vi "PM9 Set Temp and Wait.vi"(0 "VISA":refnum<visa-resource-name>="TCPIP0::169.254.70.190::502::SOCKET", 5 "Error In":errorcluster, 6 "Accuracy +/-":dbl=0.25 format="%.3g", 7 "Set Point":dbl=25.0 format="%.3g", 9 "RO(t)":bool, 11 "Min (-1 for cont.)":dbl, 12 "Refresh Rate(s)":dbl format="%#_13g", 13 "close session(t)":bool=TRUE) -> (10 "temp":sgl[](array[numeric])=[24.988047, 24.909956], 14 "visa":refnum<visa-resource-name>="TCPIP0::169.254.70.190::502::SOCKET", 15 "session out":refnum<k24>, 19 "error out":errorcluster)   [LabVIEW 2018]
uses:
  C:/RageATE-Tetra/Instruments/Ess Temp Plate/LabView Driver/Public/Watbus.dll
  Public/Watbus.dll
panel:
  out "read_loop(t)":bool
  out "sec":i32
  out "x/y":dbl
  out "vi called (t)":bool
  out "call chain":string[](array[string])
  out "soak(f)":bool=TRUE
  out "elapsed(s)":i32
  out "start":dbl=15892.4205274 format="%_19f"
  in  "Stop":bool
  out "LSL":dbl=24.75
  out "USL":dbl=25.25
  in  "deviceType":i32(ring) items=["Controller", "RUI", "PC", "CommsCard"]
  in  "InstanceId":i32=1
  in  "Zone":i32=1
  in  "TemperatureUnits":i16(ring) items=["Degrees C", "Degrees F"]
  out "Waveform Chart 3":cluster{"Value":sgl, "Value":sgl}(graph)={"Value"=24.988047, "Value"=24.909956}
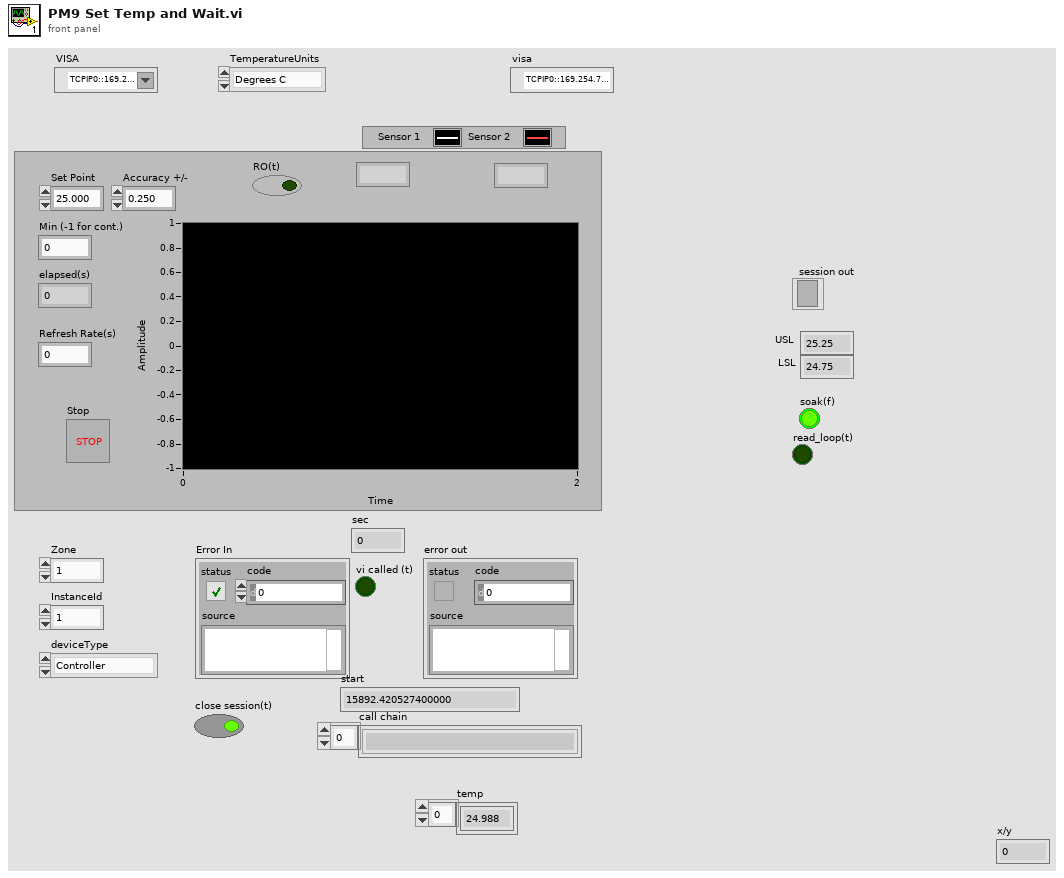
[diagram p1: front panel]
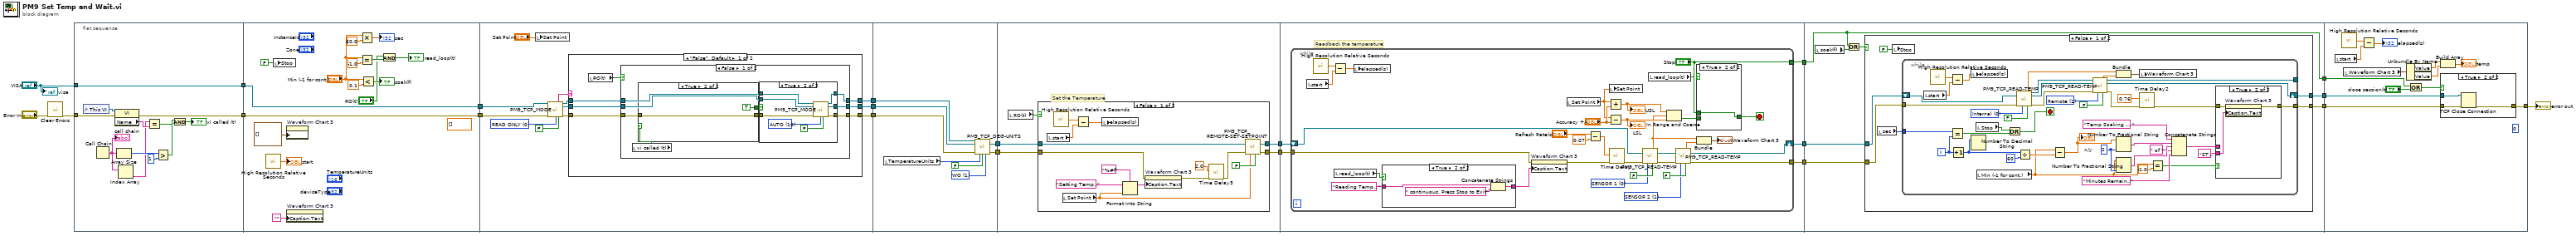
[diagram p0: block diagram]
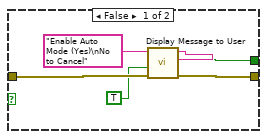
[diagram p2: hidden frame]
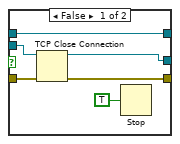
[diagram p3: hidden frame]
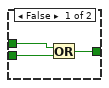
[diagram p8: hidden frame]
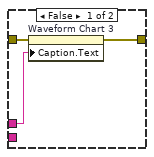
[diagram p9: hidden frame]
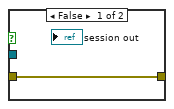
[diagram p11: hidden frame]
diagram:
  n1 = call <vilib>:"Clear Errors.vi"("error in (no error)"="Error In") -> ("error out"=w4:errorcluster)  [unwired: 5 in, 1 out]
  n2 = flat-sequence {
    tunnel: w4 -> [w23]
    tunnel: "VISA" -> [w33]
    tunnel: [w33] -> w2
    tunnel: [w22] -> w1
    tunnel: [w48] -> w15
    tunnel: [w47] -> w14
    tunnel: w2 -> [w48]
    tunnel: w1 -> [w47]
    tunnel: [w51] -> w17
    tunnel: [w57] -> w16
    tunnel: w15 -> [w56]
    tunnel: w14 -> [w59]
    tunnel: [w52] -> w6
    tunnel: [w108] -> w19
    tunnel: [w109] -> w18
    tunnel: w17 -> [w111]
    tunnel: w16 -> [w110]
    tunnel: w6 -> [w104]
    tunnel: [w114] -> w21
    tunnel: [w113] -> w20
    tunnel: w19 -> [w116]
    tunnel: w18 -> [w115]
    tunnel: [w136] -> w13
    tunnel: w21 -> [w138]
    tunnel: w20 -> [w137]
    tunnel: [w135] -> w10
    tunnel: [w134] -> w8
    tunnel: w13 -> [w182]
    tunnel: [w181] -> w12
    tunnel: [w185] -> w11
    tunnel: w10 -> [w183]
    tunnel: [w183] -> w9
    tunnel: w8 -> [w184]
    tunnel: w12 -> [w253]
    tunnel: w11 -> [w249]
    tunnel: w9 -> [w250]
    tunnel: [w241] -> w3
    frame #0 {
      n3 = control-ref of="This VI"() -> (w25:refnum<vi>)
      n4 = Call Chain() -> (call chain=w28:string[])
      "call chain" <- w28
      n5 = property class="VI"(reference=w25, error in=w23) -> (error out=w22:errorcluster, "Name"=w27:string)  [unwired: 1 out]
      n6 = Array Size(array=w28) -> (size(s)=w29:i32)
      n7 = Index Array(array=w28) -> (element=w26:string)  [unwired: 1 in]
      n8 = Equal?(x=w26, y=w27) -> (x = y?=w30:bool)
      n9 = Greater?(x=w29, y=1) -> (0:w31:bool)
      n10 = And(x=w31, y=w30) -> (x .and. y?=→"vi called (t)":bool)
    }
    frame #1 {
      (unwired) dbl[] [] ("History Data")
      n11 = call <vilib>:"High Resolution Relative Seconds.vi"() -> ("relative seconds"=→"start":dbl)
      n12 = local write "Stop"(FALSE ("Stop")) -> ()
      n13 = property on="Waveform Chart 3" class="WFChart (strict)"("History Data"=cluster{"Value":sgl, "Value":sgl}[] []) -> ()  [unwired: 2 in, 2 out]
      n14 = property on="Waveform Chart 3" class="WFChart (strict)"("Caption.Text"="") -> ()  [unwired: 2 in, 2 out]
      n15 = Multiply(x="Min (-1 for cont.)", y=60.0) -> (x*y=→"sec":dbl)
      n16 = Equal?(x="Min (-1 for cont.)", y=-1.0) -> (x = y?=w37:bool)
      n17 = Less?(x="Min (-1 for cont.)", y=0.1) -> (x < y?=→"soak(f)":bool)
      n18 = And(x="RO(t)", y=w37) -> (x .and. y?=→"read_loop(t)":bool)
    }
    frame #2 {
      w54 = u16 0 items=["READ ONLY"=0, "AUTO"=10, "OFF"=62, "MAN"=54] ("MODE")
      n19 = local write "Set Point"("Set Point") -> ()
      n20 = call "PM9_TCP_MODE.vi"("VISA"=w56, "error in (no error)"=w59, "MODE"=w54, "Close tcp(t)"=FALSE) -> ("mode(read)"=w49:string, "visa out"=w50:refnum<visa-resource-name>, "connection ID out"=w53:refnum<k5>, "error out"=w58:errorcluster)  [unwired: 8 in]
      n21 = case shown="\"False\", Default" w49 {
        tunnel: w58 -> [w67 w103]
        tunnel: [w66 w103] -> w57
        tunnel: w53 -> [w65 w102]
        tunnel: [w64 w102] -> w52
        tunnel: [w62 w101] -> w51
        tunnel: w50 -> [w63 w101]
        frame "False", Default {
          n22 = local read "RO(t)"() -> (w61:bool)
          n23 = case shown="False" w61 {
            tunnel: w67 -> [w76 w98]
            tunnel: [w74 w98] -> w66
            tunnel: w65 -> [w72 w99]
            tunnel: [w71 w99] -> w64
            tunnel: w63 -> [w70 w100]
            tunnel: [w69 w100] -> w62
            frame False {
              n24 = local read "vi called (t)"() -> (w68:bool)
              n25 = case shown="True" w68 {
                tunnel: w76 -> [w81 w82]
                tunnel: [w78 TRUE ("OK")] -> w75
                tunnel: [w77 w82] -> w73
                frame False {
                  n26 = call "Display Message to User"("error in (no error)"=w81, "Enable"=TRUE, "Message"="Enable Auto Mode (Yes)\nNo to Cancel") -> ("error out"=w77:errorcluster, "OK"=w78:bool)  [unwired: 7 in]
                }
                frame True {
                }
              }
              n27 = case shown="True" w75 {
                tunnel: [w86 w97] -> w74
                tunnel: w73 -> [w87 w96]
                tunnel: w72 -> [w88 w94]
                tunnel: [w84 w93] -> w71
                tunnel: w70 -> [w89 w92]
                tunnel: [w89 w91] -> w69
                frame False {
                  n28 = TCP Close Connection(connection ID=w88, error in (no error)=w87) -> (connection ID out=w84:refnum<k5>, error out=w86:errorcluster)  [unwired: 1 in]
                  n29 = Stop(stop? (T)=TRUE) -> ()
                }
                frame True {
                  w95 = u16 10 items=["READ ONLY"=0, "AUTO"=10, "OFF"=62, "MAN"=54] ("MODE")
                  n30 = call "PM9_TCP_MODE.vi"("VISA"=w92, "connection ID"=w94, "error in (no error)"=w96, "MODE"=w95, "Close tcp(t)"=FALSE) -> ("visa out"=w91:refnum<visa-resource-name>, "connection ID out"=w93:refnum<k5>, "error out"=w97:errorcluster)  [unwired: 7 in, 1 out]
                }
              }
            }
            frame True {
            }
          }
        }
        frame "AUTO" {
        }
      }
    }
    frame #3 {
      w107 = 1 items=["RO", "WO"] ("RO|WO")
      n31 = local read "TemperatureUnits"() -> (w106:i16)
      n32 = call "PM9_TCP_DEG-UNITS.vi"("VISA"=w111, "connection ID"=w104, "error in (no error)"=w110, "Units[C|F]"=w106, "Close TCP(t)"=FALSE, "RO|WO"=w107) -> ("connection ID out"=w109:refnum<k5>, "error out"=w108:errorcluster)  [unwired: 6 in, 2 out]
    }
    frame #4 {
      # "Set the Temperature"
      n33 = local read "RO(t)"() -> (w112:bool)
      n34 = case shown="False" w112 {
        tunnel: [w130 w132] -> w114
        tunnel: [w131 w133] -> w113
        tunnel: w116 -> [w127 w133]
        tunnel: w115 -> [w129 w132]
        frame False {
          n35 = local read "start"() -> (w117:dbl)
          n36 = call <vilib>:"High Resolution Relative Seconds.vi"() -> ("relative seconds"=w118:dbl)
          n37 = local read "Set Point"() -> (w126:dbl)
          n38 = Subtract(x=w118, y=w117) -> (x-y=w119:dbl)
          n39 = local write "elapsed(s)"(w119) -> ()
          n40 = Format Into String(format string="%#f", initial string="Setting Temp.." ("Caption.Text"), w126) -> (resulting string=w124:string)  [unwired: 1 in, 1 out]
          n41 = property on="Waveform Chart 3" class="WFChart (strict)"(error in=w127, "Caption.Text"=w124) -> (error out=w121:errorcluster)  [unwired: 1 in, 1 out]
          n42 = call "Time Delay3"("error in (no error)"=w121, "Delay Time (s)"=2.0) -> ("error out"=w122:errorcluster)  [unwired: 9 in]
          n43 = call "PM9_TCP_REMOTE-SET-SETPOINT.vi"("connection ID"=w129, "error in (no error)"=w122, "Temp"=w126, "Close TCP(t)"=FALSE) -> ("connection ID out"=w130:refnum<k5>, "error out"=w131:errorcluster)  [unwired: 9 in, 1 out]
        }
        frame True {
        }
      }
    }
    frame #5 {
      # "Readback the temperature"
      n44 = while {
        tunnel: w137 -> [w145]
        shift-right: [w160] -> w136
        shift-left: w138 -> [w154]
        tunnel: ["Stop"] -> w135
        tunnel: [w161] -> w134
        stop <- w148 stop-if-true
        w149 = u16 0 items=["SENSOR 1", "SENSOR 2"] ("Sensor")
        w150 = u16 1 items=["SENSOR 1", "SENSOR 2"] ("Sensor")
        n45 = local read "start"() -> (w139:dbl)
        n46 = call <vilib>:"High Resolution Relative Seconds.vi"() -> ("relative seconds"=w140:dbl)
        n47 = Subtract(x=w140, y=w139) -> (x-y=w141:dbl)
        n48 = local read "read_loop(t)"() -> (w142:bool)
        n49 = local write "elapsed(s)"(w141) -> ()
        n50 = case shown="True" w142 {
          tunnel: "Reading Temp..." ("Caption.Text") -> [w171 w174]
          tunnel: [w171 w173] -> w143
          frame False {
          }
          frame True {
            n51 = Concatenate Strings(w174, " continuous. Press Stop to Exit" ("string")) -> (w173:string)
          }
        }
        n52 = property on="Waveform Chart 3" class="WFChart (strict)"(error in=w145, "Caption.Text"=w143) -> (error out=w146:errorcluster)  [unwired: 1 in, 1 out]
        n53 = local read "Set Point"() -> (w155:dbl)
        n54 = Subtract(x="Refresh Rate(s)", y=0.07) -> (x-y=w168:dbl)
        n55 = Add(x=w155, y="Accuracy +/-") -> (x+y=w157:dbl)
        "USL" <- w157
        n56 = Subtract(x=w155, y="Accuracy +/-") -> (x-y=w156:dbl)
        "LSL" <- w156
        n57 = local write "Set Point"(w155) -> ()
        n58 = call "Time Delay"("error in (no error)"=w146, "Delay Time (s)"=w168) -> ("error out"=w165:errorcluster)  [unwired: 9 in]
        n59 = call "PM9_TCP_READ-TEMP.vi"("connection ID"=w154, "error in (no error)"=w165, "Sensor"=w149, "Close tcp(t)"=FALSE) -> ("Value"=w153:sgl, "connection ID out"=w163:refnum<k5>, "error out"=w162:errorcluster)  [unwired: 8 in, 1 out]
        n60 = local read "read_loop(t)"() -> (w147:bool)
        n61 = In Range and Coerce(upper limit=w157, x=w153, lower limit=w156) -> (In Range?=w170:bool)  [unwired: 1 out]
        n62 = call "PM9_TCP_READ-TEMP.vi"("connection ID"=w163, "error in (no error)"=w162, "Sensor"=w150, "Close tcp(t)"=FALSE) -> ("Value"=w152:sgl, "connection ID out"=w160:refnum<k5>, "error out"=w161:errorcluster)  [unwired: 8 in, 1 out]
        n63 = case shown="True" w147 {
          tunnel: w170 -> [w177 _]
          tunnel: "Stop" -> [w176 w178]
          tunnel: [w175 w178] -> w148
          frame False {
            n64 = Or(x=w176, y=w177) -> (x .or. y?=w175:bool)
          }
          frame True {
          }
        }
        n65 = Bundle("Value"=w153, "Value"=w152) -> (→"Waveform Chart 3":cluster{"Value":sgl, "Value":sgl})  [unwired: 1 in]
      }
    }
    frame #6 {
      n66 = local read "soak(f)"() -> (w179:bool)
      n67 = Or(x=w183, y=w179) -> (x .or. y?=w180:bool)
      n68 = case shown="False" w180 {
        tunnel: [w190 w240] -> w185
        tunnel: w184 -> [w188 w240]
        tunnel: w182 -> [w189 w239]
        tunnel: [w191 w239] -> w181
        frame False {
          n69 = local read "sec"() -> (w187:i32)
          n70 = local write "Stop"(FALSE ("Stop")) -> ()
          n71 = while {
            tunnel: [w226] -> _
            shift-right: [w223] -> w191
            shift-left: w189 -> [w222]
            tunnel: w188 -> [w221]
            tunnel: [w198] -> w190
            tunnel: w187 -> [w218]
            i -> [w214]
            stop <- w217 stop-if-true
            w203 = i16 2 ("precision (6)")
            w228 = u16 1 items=["Internal", "Remote"] ("Sensor")
            w229 = u16 0 items=["Internal", "Remote"] ("Sensor")
            n72 = local read "start"() -> (w194:dbl)
            n73 = call <vilib>:"High Resolution Relative Seconds.vi"() -> ("relative seconds"=w193:dbl)
            n74 = Subtract(x=w193, y=w194) -> (x-y=w192:dbl)
            n75 = Equal?(x=w218, y=w214) -> (x = y?=w196:bool)
            n76 = Increment(x=w214) -> (x+1=w212:i32)
            n77 = local write "elapsed(s)"(w192) -> ()
            n78 = Number To Decimal String(number=w212) -> ()  [unwired: 1 in, 1 out]
            n79 = local read "Stop"() -> (w195:bool)
            n80 = local read "Min (-1 for cont.)"() -> (w200:dbl)
            n81 = Or(x=w195, y=w196) -> (x .or. y?=w217:bool)
            n82 = call "PM9_TCP_READ-TEMP.vi"("connection ID"=w222, "error in (no error)"=w221, "Sensor"=w229, "Close tcp(t)"=FALSE) -> ("Value"=w225:sgl, "visa out"=w227:refnum<visa-resource-name>, "connection ID out"=w232:refnum<k5>, "error out"=w220:errorcluster)  [unwired: 8 in]
            n83 = Divide(x=w212, y=60) -> (x/y=w210:dbl)
            n84 = Subtract(x=w200, y=w210) -> (x-y=w209:dbl)
            "x/y" <- w209
            n85 = call "PM9_TCP_READ-TEMP.vi"("VISA"=w227, "connection ID"=w232, "error in (no error)"=w220, "Sensor"=w228, "Close tcp(t)"=FALSE) -> ("Value"=w224:sgl, "visa out"=w226:refnum<visa-resource-name>, "connection ID out"=w223:refnum<k5>, "error out"=w219:errorcluster)  [unwired: 7 in]
            n86 = Bundle("Value"=w225, "Value"=w224) -> (w199:cluster{"Value":sgl, "Value":sgl})  [unwired: 1 in]
            n87 = Number To Fractional String(number=w209, precision (6)=w203) -> (F-format string=w208:string)  [unwired: 2 in]
            n88 = Number To Fractional String(number=w200, precision (6)=w203) -> (F-format string=w206:string)  [unwired: 2 in]
            n89 = local write "Waveform Chart 3"(w199) -> ()
            n90 = call "Time Delay2"("error in (no error)"=w219, "Delay Time (s)"=0.76 ("milliseconds to wait")) -> ("error out"=w216:errorcluster)  [unwired: 9 in]
            n91 = Equal?(x=w200, y=-1.0) -> (x = y?=w202:bool)
            n92 = Concatenate Strings("Temp Soaking ... ", w208, " of " ("string"), w206, "Minutes Remain.." ("string")) -> (w204:string)
            n93 = case shown="True" w202 {
              tunnel: w216 -> [w235 w238]
              tunnel: [w234 w237] -> w198
              tunnel: w204 -> [w233 _]
              tunnel: "STOP to Cancel" ("string") -> [_ w236]
              frame False {
                n94 = property on="Waveform Chart 3" class="WFChart (strict)"(error in=w235, "Caption.Text"=w233) -> (error out=w234:errorcluster)  [unwired: 1 in, 1 out]
              }
              frame True {
                n95 = property on="Waveform Chart 3" class="WFChart (strict)"(error in=w238, "Caption.Text"=w236) -> (error out=w237:errorcluster)  [unwired: 1 in, 1 out]
              }
            }
          }
        }
        frame True {
        }
      }
    }
    frame #7 {
      (unwired) i16 0 ("Monitor")
      n96 = local read "start"() -> (w247:dbl)
      n97 = call <vilib>:"High Resolution Relative Seconds.vi"() -> ("relative seconds"=w248:dbl)
      n98 = local read "Waveform Chart 3"() -> (w245:cluster{"Value":sgl, "Value":sgl})
      n99 = Subtract(x=w248, y=w247) -> (x-y=→"elapsed(s)":dbl)
      n100 = Unbundle By Name(w245) -> ("Value"=w244:sgl, "Value"=w243:sgl)
      n101 = Or(x=w250, y="close session(t)") -> (x .or. y?=w251:bool)
      n102 = Build Array(w244, w243) -> (→"temp":sgl[])
      n103 = case shown="True" w251 {
        tunnel: w253 -> [_ w257]
        tunnel: w249 -> [w254 w256]
        tunnel: [w254 w255] -> w241
        frame False {
        }
        frame True {
          n104 = TCP Close Connection(connection ID=w257, error in (no error)=w256) -> (error out=w255:errorcluster)  [unwired: 1 in, 1 out]
        }
      }
    }
  }
  "error out" <- w3
  "visa" <- "VISA"
